vi "string_to_float.vi"(1 "Array in":string[](array[string])) -> (0 "Array out":dbl[](array[numeric]))   [LabVIEW 2015]
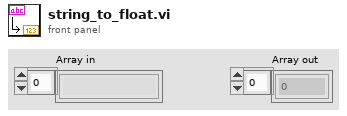
[diagram p1: front panel]
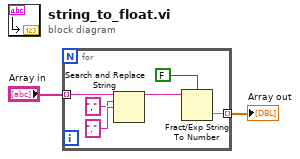
[diagram p0: block diagram]
diagram:
  n1 = for {
    tunnel: "Array in" -> [w7] mode=indexing
    tunnel: [w8] -> w1 mode=indexing
    n2 = Search and Replace String(input string=w7, search string=",", replace string="." ("replace string (\"\")")) -> (result string=w6:string)  [unwired: 5 in, 3 out]
    n3 = Fract/Exp String To Number(use system decimal point (T)=FALSE, string=w6) -> (number=w8:dbl)  [unwired: 2 in, 1 out]
  }
  "Array out" <- w1
